vi "To JSON.vi"(8 "error in (no error)":errorcluster, 10 "Path":path, 11 "DC Config in":refnum<class "DC Config.lvclass">) -> (0 "error out":errorcluster, 3 "DC Config out":refnum<class "DC Config.lvclass">)   [LabVIEW 2023, in "PXI-5441.lvlib" / "DC Config.lvclass"]
uses:
  DC Config.lvclass
  DC Config.lvclass/DC Config.ctl
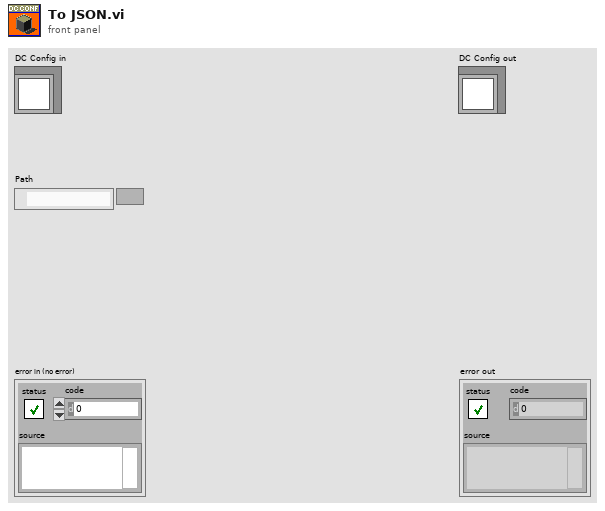
[diagram p1: front panel]
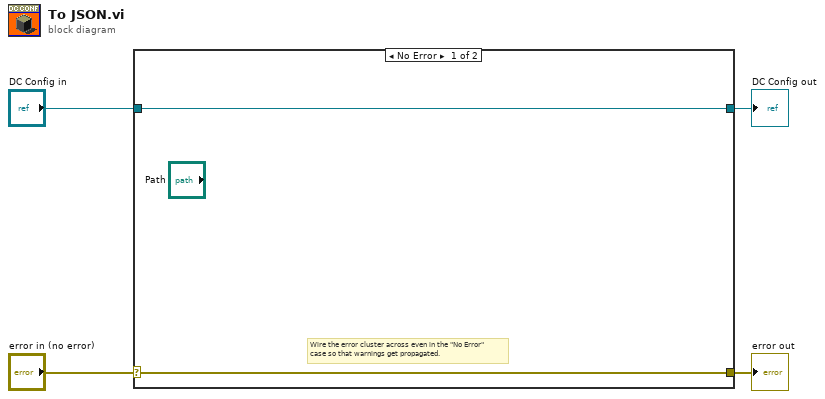
[diagram p0: block diagram]
diagram:
  n1 = case shown="No Error" "error in (no error)" {
    selector: "error in (no error)" -> [w5 w8]
    tunnel: [w5 w8] -> w3
    tunnel: [w6 w7] -> w1
    tunnel: "DC Config in" -> [w6 w7]
    frame No Error {
      # "Wire the error cluster across even in the \"No Error\"\ncase so that warnings get propagated."
    }
    frame Error {
    }
  }
  "error out" <- w3
  "DC Config out" <- w1
